vi "ThrustStand.vi"() -> ()   [LabVIEW 2023]
uses:
  <vilib>/Instr/_visa.llb/VISA Configure Serial Port (Instr).vi
panel:
  out "Power/Temperature":cluster{"RPM Out":dbl[], "Thrust Out":dbl[]}[](graph)
  out "Power":waveform(dbl)(graph)
  out "Temperature":waveform(dbl)(graph)
  out "Temperature":waveform(dbl)(graph)
  out "RPM":waveform(dbl)(graph)
  out "Thrust/Noise":cluster{"RPM Out":dbl[], "Thrust Out":dbl[]}[](graph)
  out "Thrust/Power":cluster{"RPM Out":dbl[], "Thrust Out":dbl[]}[](graph)
  in  "stop":bool
  out "RPM/Thrust":cluster{"RPM Out":dbl[], "Thrust Out":dbl[]}[](graph)
  out "Data":T1 {"Noise" scale=0.0..100.0; "Voltage" scale=0.0..25.0; "Temperature" scale=0.0..80.0; "RPM" scale=0.0..10000.0; "Thrust" scale=0.0..1000.0; "Current" scale=0.0..10.0}
  in  "Connection":T2
  out "Read":string
  out "Command":string
  in  "Control":T3={"Mode"=enum."SWEEP", "Duration"=10.0, "Sampling Rate"=10.0, "Single Mode Parameters"={"Duty Cycle"=0}, "Sweep Parameters "={"Initial Duty Cycle"=0, "Final Duty Cycle"=80, "Curve"=enum."RAMP", "Number of Steps"=0}, "Setpoint Mode Parameters"={"Value"=0.0, "Setpoint"=enum."DUTY"}, "Start"=FALSE, "Progress"=0} {"Progress" scale=0.0..100.0; "Sweep Parameters"."Final Duty Cycle" max=100; "Sweep Parameters"."Initial Duty Cycle" max=100; "Single Mode Parameters"."Duty Cycle" max=100}
  # "V"
  # "°C"
  # "A"
  # "dB"
  # "g"
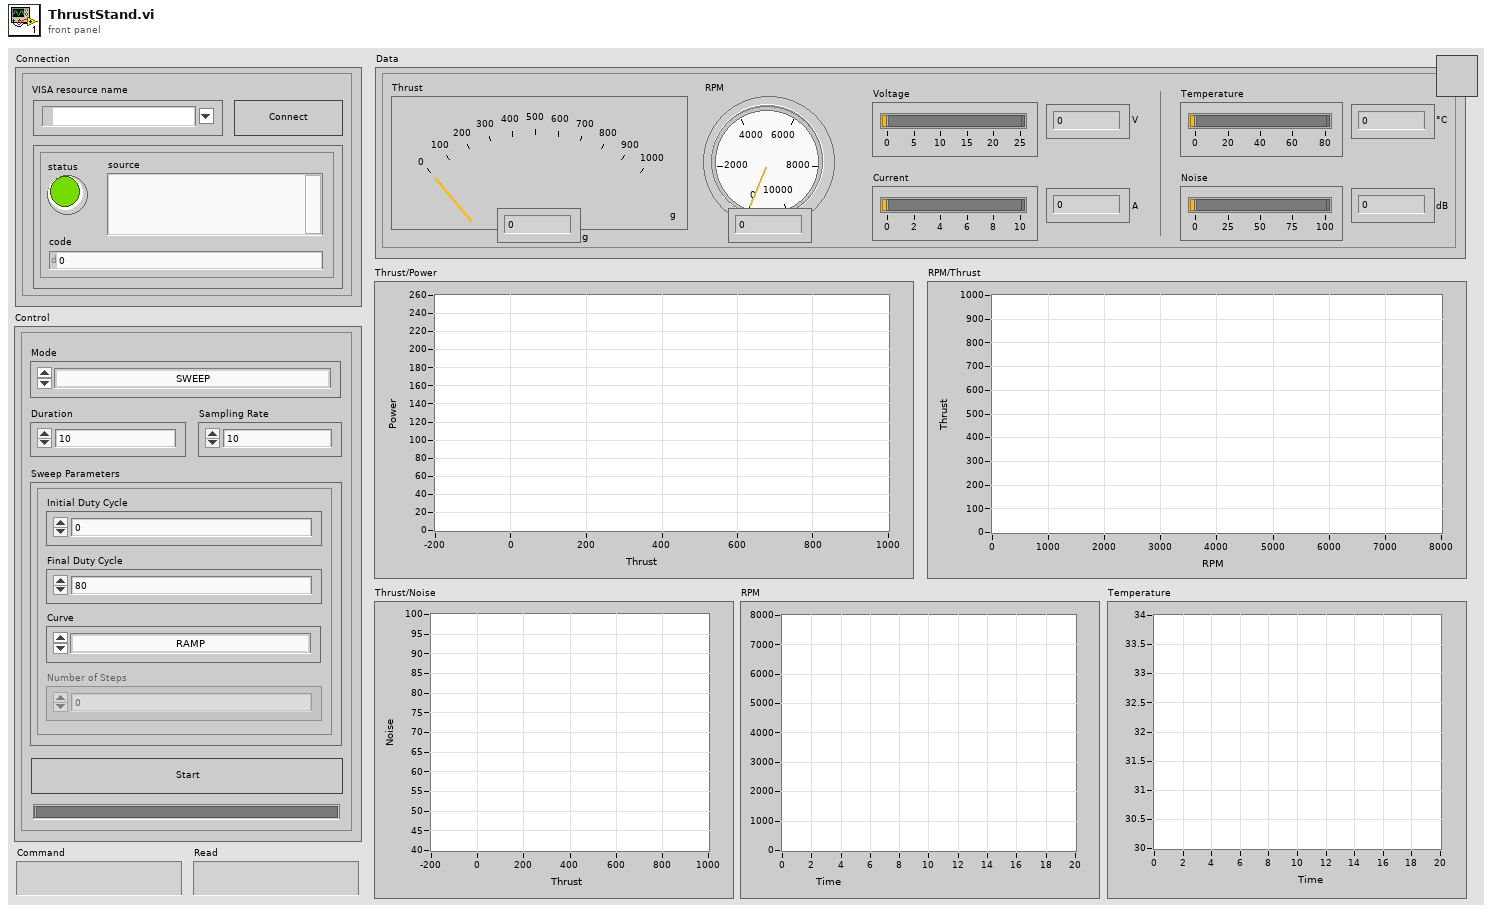
[diagram p1: front panel]
types:
  T1 = cluster{"Current":dbl, "Thrust":dbl, "RPM":dbl, "Temperature":dbl, "Voltage":dbl, "Noise":dbl, "Code":string}
  T2 = cluster{"VISA resource name":refnum<visa-resource-name>, "Connect":bool, "error out":errorcluster}
  T3 = cluster{"Mode":enum16{"SWEEP", "SETPOINT", "SINGLE"}, "Duration":dbl, "Sampling Rate":dbl, "Single Mode Parameters":cluster{"Duty Cycle":u8}, "Sweep Parameters ":cluster{"Initial Duty Cycle":u8, "Final Duty Cycle":u8, "Curve":enum16{"RAMP", "STEPS"}, "Number of Steps":u8}, "Setpoint Mode Parameters":cluster{"Value":dbl, "Setpoint":enum16{"DUTY", "RPM", "POWER", "THRUST"}}, "Start":bool, "Progress":u8}
  T4 = enum8{"Enabled", "Disabled", "Disabled and Grayed Out"}
  T5 = cluster{"Initial Duty Cycle":u8, "Final Duty Cycle":u8, "Curve":enum16{"RAMP", "STEPS"}, "Number of Steps":u8}
  T6 = cluster{"Power Out":dbl[], "Temperature Out":dbl[]}
  T7 = cluster{"Power Out":dbl[], "Temperature Out":dbl[]}[]
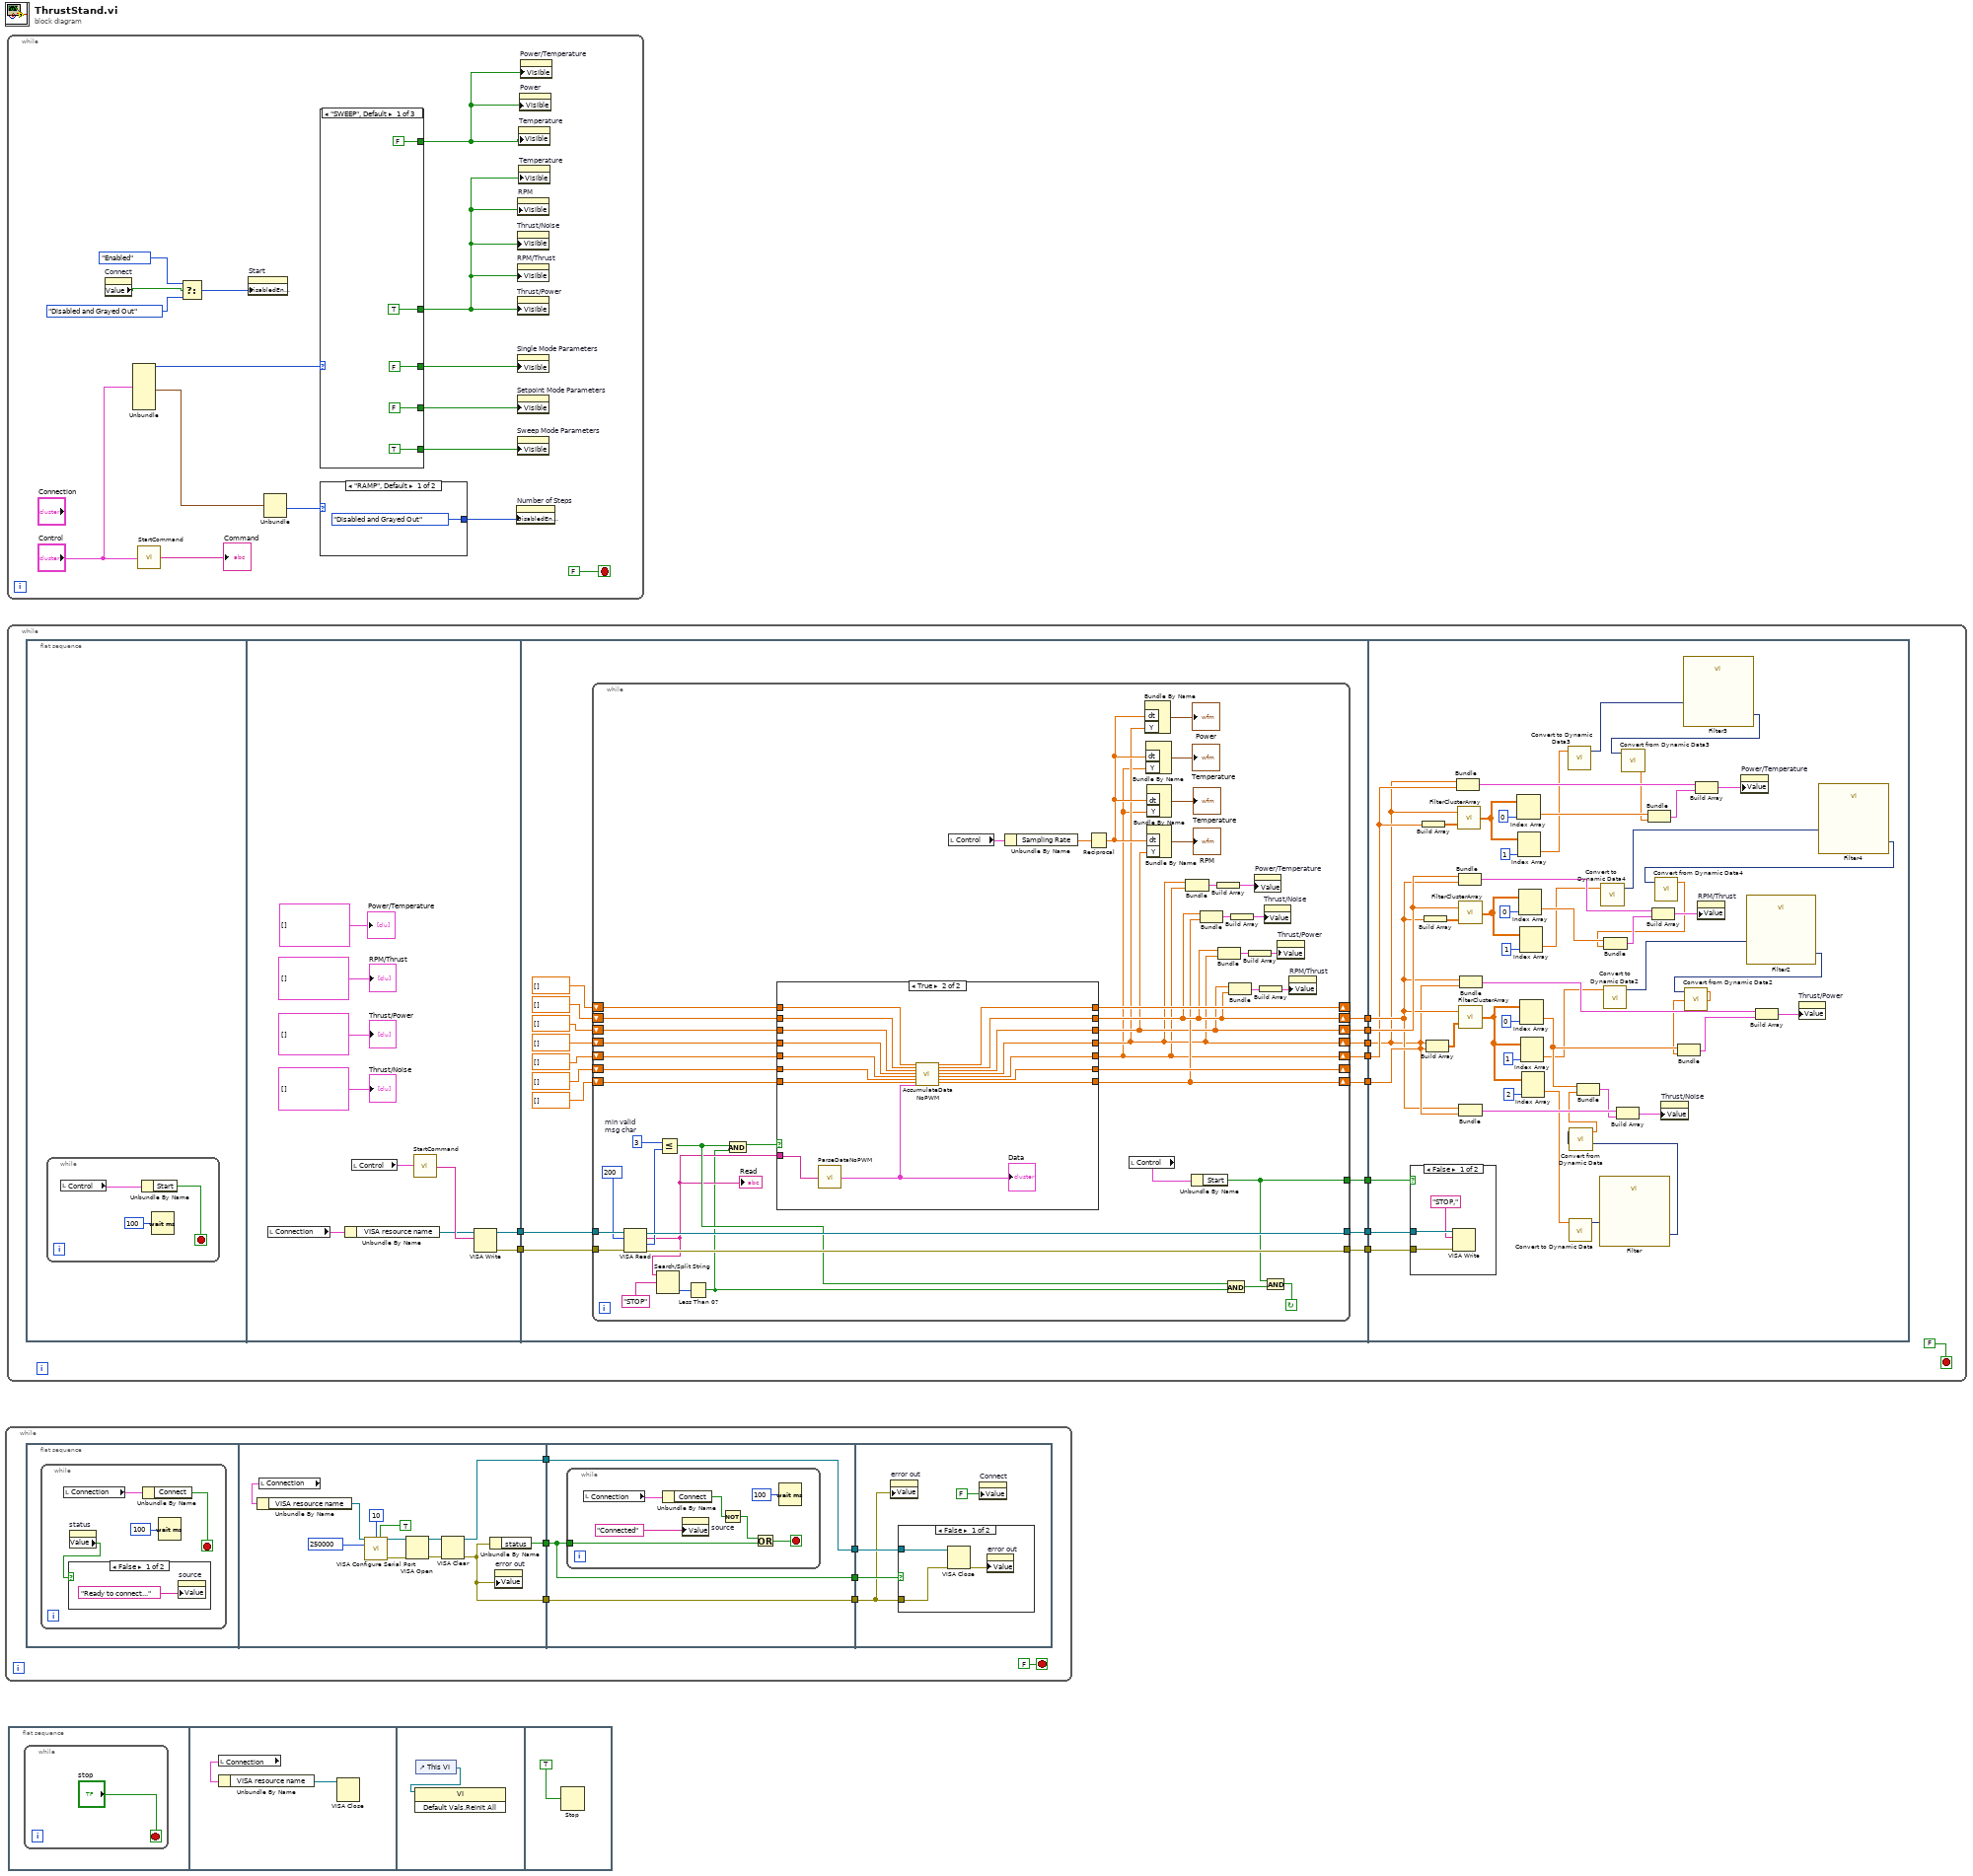
[diagram p0: block diagram]
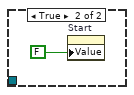
[diagram p5: hidden frame]
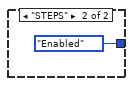
[diagram p6: hidden frame]
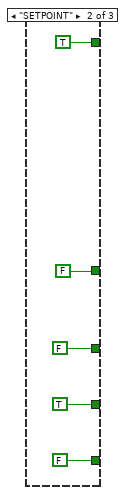
[diagram p7: hidden frame]
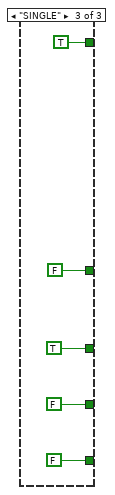
[diagram p8: hidden frame]
diagram:
  n1 = while {
    stop <- FALSE stop-if-true
    n2 = flat-sequence {
      tunnel: [w15] -> w7
      tunnel: [w14] -> w6
      tunnel: [w13] -> w5
      tunnel: w7 -> [w25]
      tunnel: [w27] -> w4
      tunnel: w6 -> [w27]
      tunnel: [w26] -> w3
      tunnel: w5 -> [w26]
      tunnel: [w25] -> w1
      tunnel: w4 -> [w37]
      tunnel: w3 -> [w35]
      tunnel: w1 -> [w36]
      frame #0 {
        n3 = while {
          stop <- w10 stop-if-true
          n4 = local read "Connection"() -> (w9:T2)
          n5 = property on="status" class="Bool (strict)"() -> ("Value"=w8:bool)  [unwired: 2 in, 2 out]
          n6 = case shown="False" w8 {
            frame False {
              n7 = property on="source" class="Str"("Value"="Ready to connect...") -> ()  [unwired: 2 in, 2 out]
            }
            frame True {
            }
          }
          n8 = Unbundle By Name(w9) -> ("Connect"=w10:bool)
          n9 = Wait (ms)(milliseconds to wait=u32 100) -> ()  [unwired: 1 out]
        }
      }
      frame #1 {
        n10 = local read "Connection"() -> (w17:T2)
        n11 = Unbundle By Name(w17) -> ("VISA resource name"=w16:refnum<visa-resource-name>)
        n12 = call-poly "VISA Configure Serial Port"("VISA resource name"=w16, "termination char\n(0xA = '\\n' = LF)"=u8 10 ("termination char\n(0xA = '\\n' = LF)"), "Enable Termination\nChar (T)"=TRUE ("Enable Termination\nChar (T)"), "baud rate (9600)"=u32 250000) -> ("VISA resource name out"=w22:refnum<visa-resource-name>, "error out"=w21:errorcluster)  [unwired: 10 in]
        n13 = VISA Open(error in (no error)=w21, VISA resource name=w22) -> (VISA resource name=w23:refnum<visa-resource-name>, error out=w24:errorcluster)  [unwired: 3 in]
        n14 = VISA Clear(VISA resource name=w23, error in (no error)=w24) -> (VISA resource name out=w14:refnum<visa-resource-name>, error out=w13:errorcluster)
        n15 = Unbundle By Name(w13) -> ("status"=w15:bool)
        n16 = property on="error out" class="Clust (strict)"("Value"=w13) -> ()  [unwired: 2 in, 2 out]
      }
      frame #2 {
        n17 = while {
          tunnel: w25 -> [w30]
          stop <- w29 stop-if-true
          n18 = local read "Connection"() -> (w33:T2)
          n19 = Unbundle By Name(w33) -> ("Connect"=w32:bool)
          n20 = property on="source" class="Str"("Value"="Connected") -> ()  [unwired: 2 in, 2 out]
          n21 = Not(x=w32) -> (.not. x?=w31:bool)
          n22 = Or(x=w31, y=w30) -> (x .or. y?=w29:bool)
          n23 = Wait (ms)(milliseconds to wait=u32 100) -> ()  [unwired: 1 out]
        }
      }
      frame #3 {
        n24 = property on="error out" class="Clust (strict)"("Value"=w35) -> ()  [unwired: 2 in, 2 out]
        n25 = case shown="False" w36 {
          tunnel: w37 -> [w41 _]
          tunnel: w35 -> [w40 _]
          frame False {
            n26 = VISA Close(VISA resource name=w41, error in (no error)=w40) -> (error out=w39:errorcluster)
            n27 = property on="error out" class="Clust (strict)"("Value"=w39) -> ()  [unwired: 2 in, 2 out]
          }
          frame True {
          }
        }
        n28 = property on="Connect" class="Bool (strict)"("Value"=FALSE) -> ()  [unwired: 2 in, 2 out]
      }
    }
  }
  n29 = while {
    stop <- FALSE stop-if-true
    n30 = property on="Connect" class="Bool (strict)"() -> ("Value"=w45:bool)  [unwired: 2 in, 2 out]
    n31 = Unbundle("Control") -> ("Mode"=w51:enum16{"SWEEP", "SETPOINT", "SINGLE"}, "Sweep Parameters"=w52:T5)  [unwired: 6 out]
    n32 = call "StartCommand.vi"("Control"="Control") -> ("String"=→"Command":string)
    n33 = Select(t=T4."Enabled" ("Disabled"), s=w45, f=T4."Disabled and Grayed Out" ("Disabled")) -> (s? t:f=w46:T4)
    n34 = property on="Start" class="Bool (strict)"("DisabledEnum"=w46) -> ()  [unwired: 2 in, 2 out]
    n35 = Unbundle(w52) -> ("Curve"=w54:enum16{"RAMP", "STEPS"})  [unwired: 3 out]
    n36 = case shown="\"SWEEP\", Default" w51 {
      tunnel: [FALSE ("Visible") FALSE ("Visible") TRUE ("Visible")] -> w57
      tunnel: [TRUE ("Visible") FALSE ("Visible") FALSE ("Visible")] -> w56
      tunnel: [FALSE ("Visible") TRUE ("Visible") FALSE ("Visible")] -> w55
      tunnel: [TRUE ("Visible") FALSE ("Visible") FALSE ("Visible")] -> w43
      tunnel: [FALSE ("Visible") TRUE ("Visible") TRUE ("Visible")] -> w42
      frame "SWEEP", Default {
      }
      frame "SETPOINT" {
      }
      frame "SINGLE" {
      }
    }
    n37 = case shown="\"RAMP\", Default" w54 {
      tunnel: [T4."Disabled and Grayed Out" ("DisabledEnum") T4."Enabled" ("DisabledEnum")] -> w53
      frame "RAMP", Default {
      }
      frame "STEPS" {
      }
    }
    n38 = property on="Number of Steps" class="DigNum (strict)"("DisabledEnum"=w53) -> ()  [unwired: 2 in, 2 out]
    n39 = property on="Thrust/Noise" class="XYGraph (strict)"("Visible"=w43) -> ()  [unwired: 2 in, 2 out]
    n40 = property on="RPM/Thrust" class="XYGraph (strict)"("Visible"=w43) -> ()  [unwired: 2 in, 2 out]
    n41 = property on="Thrust/Power" class="XYGraph (strict)"("Visible"=w43) -> ()  [unwired: 2 in, 2 out]
    n42 = property on="Single Mode Parameters" class="Clust (strict)"("Visible"=w57) -> ()  [unwired: 2 in, 2 out]
    n43 = property on="Setpoint Mode Parameters" class="Clust (strict)"("Visible"=w55) -> ()  [unwired: 2 in, 2 out]
    n44 = property on="Sweep Mode Parameters" class="Clust (strict)"("Visible"=w56) -> ()  [unwired: 2 in, 2 out]
    n45 = property on="RPM" class="WFGraph (strict)"("Visible"=w43) -> ()  [unwired: 2 in, 2 out]
    n46 = property on="Temperature" class="WFGraph (strict)"("Visible"=w42) -> ()  [unwired: 2 in, 2 out]
    n47 = property on="Temperature" class="WFGraph (strict)"("Visible"=w43) -> ()  [unwired: 2 in, 2 out]
    n48 = property on="Power" class="WFGraph (strict)"("Visible"=w42) -> ()  [unwired: 2 in, 2 out]
    n49 = property on="Power/Temperature" class="XYGraph (strict)"("Visible"=w42) -> ()  [unwired: 2 in, 2 out]
  }
  n50 = while {
    stop <- FALSE stop-if-true
    n51 = flat-sequence {
      tunnel: [w97] -> w81
      tunnel: [w96] -> w80
      tunnel: [w113] -> w85
      tunnel: [w112] -> w84
      tunnel: [w111] -> w83
      tunnel: w80 -> [w114]
      tunnel: w81 -> [w115]
      tunnel: [w106] -> w79
      tunnel: [w105] -> w78
      tunnel: [w101] -> w77
      tunnel: [w100] -> w76
      tunnel: [w99] -> w75
      tunnel: w85 -> [w236]
      tunnel: w84 -> [w235]
      tunnel: w83 -> [w234]
      tunnel: w79 -> [w230]
      tunnel: w78 -> [w214]
      tunnel: w77 -> [w197]
      tunnel: w76 -> [w215]
      tunnel: w75 -> [w198]
      frame #0 {
        n52 = while {
          stop <- w87 stop-if-true
          n53 = local read "Control"() -> (w86:T3)
          n54 = Unbundle By Name(w86) -> ("Start"=w87:bool)
          n55 = Wait (ms)(milliseconds to wait=u32 100) -> ()  [unwired: 1 out]
        }
      }
      frame #1 {
        n56 = local read "Connection"() -> (w93:T2)
        n57 = Unbundle By Name(w93) -> ("VISA resource name"=w94:refnum<visa-resource-name>)
        n58 = local read "Control"() -> (w95:T3)
        n59 = call "StartCommand.vi"("Control"=w95) -> ("String"=w98:string)
        n60 = VISA Write(VISA resource name=w94, write buffer=w98) -> (VISA resource name out=w97:refnum<visa-resource-name>, error out=w96:errorcluster)  [unwired: 1 in, 1 out]
        "RPM/Thrust" <- cluster{"RPM Out":dbl[], "Thrust Out":dbl[]}[] [] ("appended array")
        "Thrust/Power" <- cluster{"RPM Out":dbl[], "Thrust Out":dbl[]}[] [] ("appended array")
        "Thrust/Noise" <- cluster{"RPM Out":dbl[], "Thrust Out":dbl[]}[] [] ("appended array")
        "Power/Temperature" <- cluster{"RPM Out":dbl[], "Thrust Out":dbl[]}[] [] ("appended array")
      }
      frame #2 {
        n61 = while {
          tunnel: w115 -> [w161]
          tunnel: w114 -> [w160]
          tunnel: [w158] -> w113
          tunnel: [w157] -> w112
          tunnel: [w153] -> w111
          shift-right: [w128] -> w100
          shift-left: dbl[] [] -> [w149]
          shift-right: [w147] -> _
          shift-left: dbl[] [] -> [w148]
          shift-right: [w116] -> w99
          shift-left: dbl[] [] -> [w146]
          shift-right: [w117] -> w101
          shift-left: dbl[] [] -> [w140]
          shift-right: [w124] -> w106
          shift-left: dbl[] [] -> [w139]
          shift-right: [w129] -> w105
          shift-left: dbl[] [] -> [w138]
          shift-right: [w137] -> _
          shift-left: dbl[] [] -> [w136]
          stop <- w159 continue-if-true
          w154 = u32 3  # min valid msg char
          n62 = VISA Read(VISA resource name=w161, byte count=u32 200, error in (no error)=w160) -> (VISA resource name out=w158:refnum<visa-resource-name>, read buffer=w144:string, return count=w155:u32, error out=w157:errorcluster)
          "Read" <- w144
          n63 = Search/Split String(string=w144, search string/char (-)="STOP") -> (offset of match=w142:i32)  [unwired: 1 in, 2 out]
          n64 = Less Or Equal?(x=w154, y=w155) -> (x <= y?=w150:bool)
          n65 = Less Than 0?(x=w142) -> (x < 0?=w141:bool)
          n66 = And(x=w150, y=w141) -> (x .and. y?=w143:bool)
          n67 = case shown="True" w143 {
            tunnel: w144 -> [_ w184]
            tunnel: w149 -> [w166 w182]
            tunnel: [w166 w179] -> w128
            tunnel: w148 -> [w167 w181]
            tunnel: [w167 w178] -> w147
            tunnel: w146 -> [w168 w180]
            tunnel: [w168 w177] -> w116
            tunnel: [w165 w176] -> w117
            tunnel: w140 -> [w165 w175]
            tunnel: [w164 w174] -> w124
            tunnel: w139 -> [w164 w173]
            tunnel: [w163 w172] -> w129
            tunnel: w138 -> [w163 w171]
            tunnel: [w162 w170] -> w137
            tunnel: w136 -> [w162 w169]
            frame False {
            }
            frame True {
              n68 = call "ParseDataNoPWM.vi"("input string"=w184) -> ("output cluster"=w183:T1)
              "Data" <- w183
              n69 = call "AccumulateDataNoPWM.vi"("Current In"=w169, "Thrust In"=w171, "RPM In"=w173, "Power In"=w175, "Temperature In"=w180, "Voltage In"=w181, "Noise In"=w182, "Data"=w183) -> ("Current Out"=w170:dbl[], "Thrust Out"=w172:dbl[], "RPM Out"=w174:dbl[], "Power Out"=w176:dbl[], "Temperature Out"=w177:dbl[], "Voltage Out"=w178:dbl[], "Noise Out"=w179:dbl[])  [unwired: 13 in]
            }
          }
          n70 = local read "Control"() -> (w126:T3)
          n71 = Unbundle By Name(w126) -> ("Sampling Rate"=w127:dbl)
          n72 = Reciprocal(x=w127) -> (1/x=w120:dbl)
          n73 = local read "Control"() -> (w151:T3)
          n74 = Bundle By Name("dt"=w120, "Y"=w117) -> (→"Power":waveform(dbl))  [unwired: 1 in]
          n75 = Bundle By Name("dt"=w120, "Y"=w116) -> (→"Temperature":waveform(dbl))  [unwired: 1 in]
          n76 = Bundle By Name("dt"=w120, "Y"=w116) -> (→"Temperature":waveform(dbl))  [unwired: 1 in]
          n77 = Bundle By Name("dt"=w120, "Y"=w124) -> (→"RPM":waveform(dbl))  [unwired: 1 in]
          n78 = Bundle("Power Out"=w117, "Temperature Out"=w116) -> (w119:T6)  [unwired: 1 in]
          n79 = Unbundle By Name(w151) -> ("Start"=w153:bool)
          n80 = Bundle("Thrust Out"=w129, "Noise Out"=w128) -> (w131:cluster{"Thrust Out":dbl[], "Noise Out":dbl[]})  [unwired: 1 in]
          n81 = Build Array(w119) -> (w118:T7)
          n82 = Bundle("Thrust Out"=w129, "Power Out"=w117) -> (w133:cluster{"Thrust Out":dbl[], "Power Out":dbl[]})  [unwired: 1 in]
          n83 = And(x=w150, y=w141) -> (x .and. y?=w152:bool)
          n84 = Bundle("RPM Out"=w124, "Thrust Out"=w129) -> (w135:cluster{"RPM Out":dbl[], "Thrust Out":dbl[]})  [unwired: 1 in]
          n85 = Build Array(w131) -> (w130:cluster{"Thrust Out":dbl[], "Noise Out":dbl[]}[])
          n86 = Build Array(w133) -> (w132:cluster{"Thrust Out":dbl[], "Power Out":dbl[]}[])
          n87 = property on="Power/Temperature" class="XYGraph (strict)"("Value"=w118) -> ()  [unwired: 2 in, 2 out]
          n88 = Build Array(w135) -> (w134:cluster{"RPM Out":dbl[], "Thrust Out":dbl[]}[])
          n89 = property on="Thrust/Noise" class="XYGraph (strict)"("Value"=w130) -> ()  [unwired: 2 in, 2 out]
          n90 = And(x=w153, y=w152) -> (x .and. y?=w159:bool)
          n91 = property on="Thrust/Power" class="XYGraph (strict)"("Value"=w132) -> ()  [unwired: 2 in, 2 out]
          n92 = property on="RPM/Thrust" class="XYGraph (strict)"("Value"=w134) -> ()  [unwired: 2 in, 2 out]
        }
      }
      frame #3 {
        n93 = case shown="False" w234 {
          tunnel: w236 -> [w239 _]
          tunnel: w235 -> [w238 _]
          frame False {
            n94 = VISA Write(VISA resource name=w239, write buffer="STOP,", error in (no error)=w238) -> ()  [unwired: 3 out]
          }
          frame True {
            n95 = property on="Start" class="Bool (strict)"("Value"=FALSE) -> ()  [unwired: 2 in, 2 out]
          }
        }
        n96 = Build Array(w198) -> (w207:dbl[][])
        n97 = Build Array(w214) -> (w226:dbl[][])
        n98 = Build Array(w197, w215) -> (w224:dbl[][])
        n99 = Bundle(w197, w198) -> (w206:cluster{dbl[], dbl[]})  [unwired: 1 in]
        n100 = call "FilterClusterArray.vi"("Ys IN"=w207, "X IN"=w197) -> ("OUT"=w210:dbl[][])
        n101 = Bundle(w230, w214) -> (w225:cluster{dbl[], dbl[]})  [unwired: 1 in]
        n102 = call "FilterClusterArray.vi"("Ys IN"=w226, "X IN"=w230) -> ("OUT"=w231:dbl[][])
        n103 = call "FilterClusterArray.vi"("Ys IN"=w224, "X IN"=w214) -> ("OUT"=w220:dbl[][])
        n104 = Bundle(w214, w215) -> (w204:cluster{dbl[], dbl[]})  [unwired: 1 in]
        n105 = Bundle(w214, w197) -> (w217:cluster{dbl[], dbl[]})  [unwired: 1 in]
        n106 = Index Array(array=w210, index (col)=0) -> (element=w209:dbl[])  [unwired: 1 in]
        n107 = Index Array(array=w210, index (col)=1) -> (element=w190:dbl[])  [unwired: 1 in]
        n108 = Index Array(array=w231, index (col)=0) -> (element=w229:dbl[])  [unwired: 1 in]
        n109 = Index Array(array=w231, index (col)=1) -> (element=w186:dbl[])  [unwired: 1 in]
        n110 = Index Array(array=w220, index (col)=0) -> (element=w219:dbl[])  [unwired: 1 in]
        n111 = Index Array(array=w220, index (col)=1) -> (element=w194:dbl[])  [unwired: 1 in]
        n112 = Index Array(array=w220, index (col)=2) -> (element=w202:dbl[])  [unwired: 1 in]
        n113 = call "Convert to Dynamic Data3"("Array"=w190) -> ("Dynamic Data Type"=w192:dynamicdata)  [unwired: 3 in]
        n114 = call "Convert to Dynamic Data"("Array"=w202) -> ("Dynamic Data Type"=w201:dynamicdata)  [unwired: 3 in]
        n115 = call "Filter"("Signal"=w201) -> ("Filtered Signal"=w200:dynamicdata)  [unwired: 9 in, 1 out]
        n116 = call "Convert from Dynamic Data"("Dynamic Data Type"=w200) -> ("Array"=w199:dbl[])  [unwired: 3 in]
        n117 = Bundle("OUT"=w219, "Array"=w199) -> (w203:cluster{"OUT":dbl[], "Array":dbl[]})  [unwired: 1 in]
        n118 = call "Convert to Dynamic Data4"("Array"=w186) -> ("Dynamic Data Type"=w188:dynamicdata)  [unwired: 3 in]
        n119 = call "Convert to Dynamic Data2"("Array"=w194) -> ("Dynamic Data Type"=w196:dynamicdata)  [unwired: 3 in]
        n120 = Build Array(w204, w203) -> (w213:cluster{"OUT":dbl[], "Array":dbl[]}[])
        n121 = property on="Thrust/Noise" class="XYGraph (strict)"("Value"=w213) -> ()  [unwired: 2 in, 2 out]
        n122 = call "Filter3"("Signal"=w192) -> ("Filtered Signal"=w191:dynamicdata)  [unwired: 9 in, 1 out]
        n123 = call "Convert from Dynamic Data3"("Dynamic Data Type"=w191) -> ("Array"=w189:dbl[])  [unwired: 3 in]
        n124 = Bundle("OUT"=w209, "Array"=w189) -> (w208:cluster{"OUT":dbl[], "Array":dbl[]})  [unwired: 1 in]
        n125 = Build Array(w206, w208) -> (w205:cluster{"OUT":dbl[], "Array":dbl[]}[])
        n126 = property on="Power/Temperature" class="XYGraph (strict)"("Value"=w205) -> ()  [unwired: 2 in, 2 out]
        n127 = call "Filter2"("Signal"=w196) -> ("Filtered Signal"=w195:dynamicdata)  [unwired: 9 in, 1 out]
        n128 = call "Convert from Dynamic Data2"("Dynamic Data Type"=w195) -> ("Array"=w193:dbl[])  [unwired: 3 in]
        n129 = Bundle("OUT"=w219, "Array"=w193) -> (w216:cluster{"OUT":dbl[], "Array":dbl[]})  [unwired: 1 in]
        n130 = Build Array(w217, w216) -> (w218:cluster{"OUT":dbl[], "Array":dbl[]}[])
        n131 = property on="Thrust/Power" class="XYGraph (strict)"("Value"=w218) -> ()  [unwired: 2 in, 2 out]
        n132 = call "Filter4"("Signal"=w188) -> ("Filtered Signal"=w187:dynamicdata)  [unwired: 9 in, 1 out]
        n133 = call "Convert from Dynamic Data4"("Dynamic Data Type"=w187) -> ("Array"=w185:dbl[])  [unwired: 3 in]
        n134 = Bundle("OUT"=w229, "Array"=w185) -> (w228:cluster{"OUT":dbl[], "Array":dbl[]})  [unwired: 1 in]
        n135 = Build Array(w225, w228) -> (w227:cluster{"OUT":dbl[], "Array":dbl[]}[])
        n136 = property on="RPM/Thrust" class="XYGraph (strict)"("Value"=w227) -> ()  [unwired: 2 in, 2 out]
      }
    }
  }
  n137 = flat-sequence {
    frame #0 {
      n138 = while {
        stop <- "stop" stop-if-true
      }
    }
    frame #1 {
      n139 = local read "Connection"() -> (w243:T2)
      n140 = Unbundle By Name(w243) -> ("VISA resource name"=w242:refnum<visa-resource-name>)
      n141 = VISA Close(VISA resource name=w242) -> ()  [unwired: 1 in, 1 out]
    }
    frame #2 {
      n142 = control-ref of="This VI"() -> (w244:refnum<vi>)
      n143 = invoke class="VI" method="Default Vals.Reinit All"(reference=w244) -> ()  [unwired: 2 in, 3 out]
    }
    frame #3 {
      n144 = Stop(stop? (T)=TRUE) -> ()
    }
  }
